vi "Build AvailableUARTs.vi"() -> ()   [LabVIEW 2020, in "CTI-Tools.lvlib"]
uses:
  CTI-Tools.lvlib
  CTI/Available UART.ctl
  CTI/UART Number.ctl
  CTI/GPIO Number.ctl
  CTI/Available AI.ctl
  CTI/ADC Number.ctl
  CTI/Available I2C.ctl
  CTI/I2C Number.ctl
  CTI/Available SPI.ctl
  CTI/SPI Number.ctl
  21cab0c9-25c6-4ca9-b5e6-ee4fa980bc66.vi
  ee84e38d-a22b-4e15-8274-eefe8c74db67.vi
  7e72eeef-3768-44c5-b0dc-33f1e46b57fc.vi
  90c1e754-4c4f-49ee-81d9-a6cb34ea2190.vi
  e62ebf84-dc5b-4819-b9da-597b06c2aefd.vi
  1b55e33d-2187-4cbe-8b8e-452fa5026134.vi
  <vilib>/AdvancedString/1D String Array to Delimited String.vi
  CTI/CTI.lvlib
panel:
  out "SPI Source":string="// Generated with CTI-Tools.lvlib\nLVBlock availableSPIs = { 45,\n    { 0x00, 0x00, 0x00, 0x02, 0x00, 0x00, 0x00, 0x00, 0x03, 0x03, 0x07, 0x13, 0x00, 0x00, 0x00, 0x03, 0x00, 0x04, 0x10, 0x00, 0x00, 0x00, 0x03, 0x02, 0x06, 0x12, 0x01, 0x00, 0x00, 0x00, 0x02, 0x0B, 0x0F, 0x00, 0x00, 0x00, 0x02, 0x08, 0x0C, 0x00, 0x00, 0x00, 0x02, 0x0A, 0x0E }\n};"
  in  "SPIs Name":string="availableSPIs"
  in  "Available SPI":T1[](array[typedef])=[{"SPI #"=0, "TX GPIOs"=[3, 7, 19], "RX GPIOs"=[0, 4, 16], "SCK GPIOs"=[2, 6, 18]}, {"SPI #"=1, "TX GPIOs"=[11, 15], "RX GPIOs"=[8, 12], "SCK GPIOs"=[10, 14]}]
  in  "I2Cs Name":string="availableI2Cs"
  out "I2C Source":string="// Generated with CTI-Tools.lvlib\nLVBlock availableI2Cs = { 44,\n    { 0x00, 0x00, 0x00, 0x02, 0x00, 0x00, 0x00, 0x00, 0x05, 0x01, 0x09, 0x0D, 0x11, 0x15, 0x00, 0x00, 0x00, 0x05, 0x00, 0x08, 0x0C, 0x10, 0x14, 0x01, 0x00, 0x00, 0x00, 0x06, 0x03, 0x07, 0x0B, 0x0F, 0x13, 0x1B, 0x00, 0x00, 0x00, 0x06, 0x02, 0x06, 0x0A, 0x0E, 0x12, 0x1A }\n};"
  in  "I2Cs":T4[](array[typedef])=[{"I2C #"=0, "SCL GPIOs"=[1, 9, 13, 17, 21], "SDA GPIOs"=[0, 8, 12, 16, 20]}, {"I2C #"=1, "SCL GPIOs"=[3, 7, 11, 15, 19, 27], "SDA GPIOs"=[2, 6, 10, 14, 18, 26]}]
  out "PWM Source":string="// Generated with CTI-Tools.lvlib\nLVBlock availablePWMs = { 18,\n    { 0x00, 0x00, 0x00, 0x0E, 0x00, 0x02, 0x04, 0x06, 0x08, 0x0A, 0x0C, 0x0E, 0x10, 0x12, 0x14, 0x16, 0x1A, 0x1C }\n};"
  in  "PWMs":T3[](array[typedef])=[0, 2, 4, 6, 8, 10, 12, 14, 16, 18, 20, 22, 26, 28]
  in  "PWM Name":string="availablePWMs"
  out "AI Source":string="// Generated with CTI-Tools.lvlib\nLVBlock availableAIs = { 10,\n    { 0x00, 0x00, 0x00, 0x03, 0x00, 0x1A, 0x01, 0x1B, 0x02, 0x1C }\n};"
  in  "AI Name":string="availableAIs"
  in  "AIs":T6[](array[typedef])=[{"ADC #"=0, "GPIO #"=26}, {"ADC #"=1, "GPIO #"=27}, {"ADC #"=2, "GPIO #"=28}]
  out "GPIO Source":string="// Generated with CTI-Tools.lvlib\nLVBlock availableGPIOs = { 30,\n    { 0x00, 0x00, 0x00, 0x1A, 0x00, 0x01, 0x02, 0x03, 0x04, 0x05, 0x06, 0x07, 0x08, 0x09, 0x0A, 0x0B, 0x0C, 0x0D, 0x0E, 0x0F, 0x10, 0x11, 0x12, 0x13, 0x14, 0x15, 0x16, 0x1A, 0x1B, 0x1C }\n};"
  in  "GPIOs":T3[](array[typedef])=[0, 1, 2, 3, 4, 5, 6, 7, 8, 9, 10, 11, 12, 13, 14, 15, 16, 17, 18, 19, 20, 21, 22, 26, 27, 28]
  in  "GPIO Name":string="availableGPIOs"
  in  "Uarts Name":string="availableUARTs"
  in  "UARTS":T8[](array[typedef])=[{"UART #"=0, "TX GPIOs"=[0, 12, 16], "RX GPIOs"=[1, 13, 17]}, {"UART #"=1, "TX GPIOs"=[4, 8], "RX GPIOs"=[5, 9]}]
  out "UART Source":string="// Generated with CTI-Tools.lvlib\nLVBlock availableUARTs = { 32,\n    { 0x00, 0x00, 0x00, 0x02, 0x00, 0x00, 0x00, 0x00, 0x03, 0x00, 0x0C, 0x10, 0x00, 0x00, 0x00, 0x03, 0x01, 0x0D, 0x11, 0x01, 0x00, 0x00, 0x00, 0x02, 0x04, 0x08, 0x00, 0x00, 0x00, 0x02, 0x05, 0x09 }\n};"
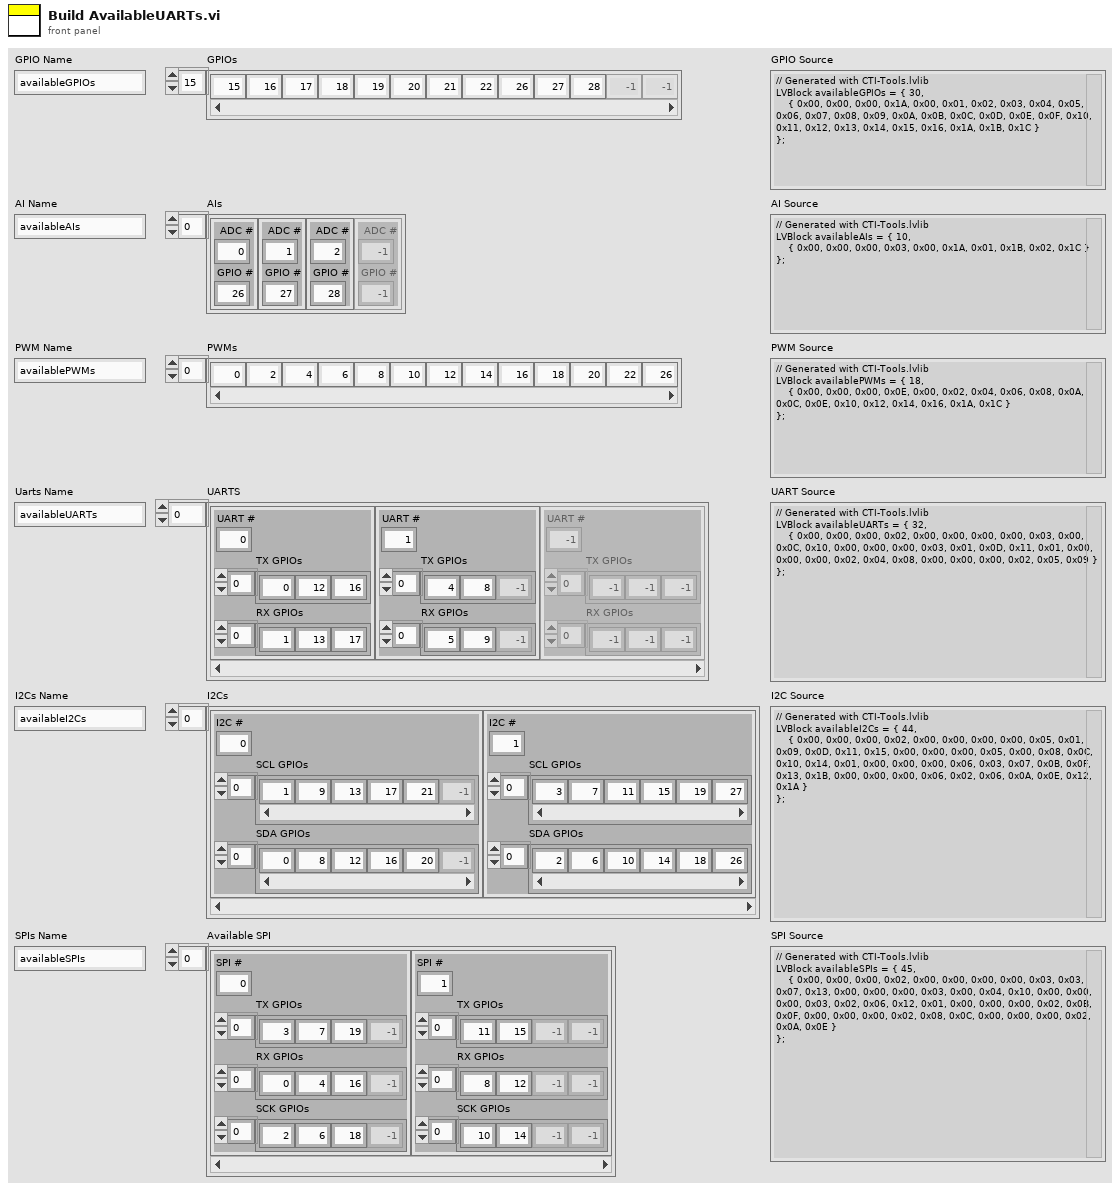
[diagram p1: front panel]
types:
  T1 = typedef "CTI.lvlib/Available SPI.ctl" = cluster{"SPI #":T2, "TX GPIOs":T3[], "RX GPIOs":T3[], "SCK GPIOs":T3[]}
  T2 = typedef "CTI.lvlib/SPI Number.ctl" = i8
  T3 = typedef "CTI.lvlib/GPIO Number.ctl" = i8
  T4 = typedef "CTI.lvlib/Available I2C.ctl" = cluster{"I2C #":T5, "SCL GPIOs":T3[], "SDA GPIOs":T3[]}
  T5 = typedef "CTI.lvlib/I2C Number.ctl" = i8
  T6 = typedef "CTI.lvlib/Available AI.ctl" = cluster{"ADC #":T7, "GPIO #":T3}
  T7 = typedef "CTI.lvlib/ADC Number.ctl" = i8
  T8 = typedef "CTI.lvlib/Available UART.ctl" = cluster{"UART #":T9, "TX GPIOs":T3[], "RX GPIOs":T3[]}
  T9 = typedef "CTI.lvlib/UART Number.ctl" = i8
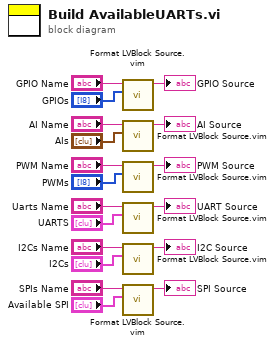
[diagram p0: block diagram]
diagram:
  n1 = call "Format LVBlock Source.vim"("Value"="GPIOs", "Name"="GPIO Name") -> ("Source"=→"GPIO Source":string)  [unwired: 9 in]
  n2 = call "Format LVBlock Source.vim"("Value"="AIs", "Name"="AI Name") -> ("Source"=→"AI Source":string)  [unwired: 9 in]
  n3 = call "Format LVBlock Source.vim"("Value"="PWMs", "Name"="PWM Name") -> ("Source"=→"PWM Source":string)  [unwired: 9 in]
  n4 = call "Format LVBlock Source.vim"("Value"="UARTS", "Name"="Uarts Name") -> ("Source"=→"UART Source":string)  [unwired: 9 in]
  n5 = call "Format LVBlock Source.vim"("Value"="I2Cs", "Name"="I2Cs Name") -> ("Source"=→"I2C Source":string)  [unwired: 9 in]
  n6 = call "Format LVBlock Source.vim"("Value"="Available SPI", "Name"="SPIs Name") -> ("Source"=→"SPI Source":string)  [unwired: 9 in]
